vi "Create HDF5 chunked dataset.vi"   [LabVIEW 2013]
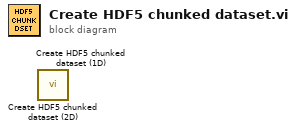
[diagram p0: block diagram]
diagram:
  n1 = call "Create HDF5 chunked dataset (2D).vi"() -> ()  [unwired: 10 in, 2 out]
  n2 = call "Create HDF5 chunked dataset (1D).vi"() -> ()  [unwired: 10 in, 2 out]
